vi "motorJoystickcore.vi"(4 "button info":T2, 6 "axis info":T1, 8 "error in":errorcluster[](array[cluster]), 9 "Motor Limits":T3, 10 "Array in":refnum<k7>[](array[refnum]), 11 "Motor serial numbers":i32[](array[numeric])) -> (0 "error out":errorcluster[](array[cluster]), 2 "XYZ position":sgl[](array[numeric]))   [LabVIEW 2014]
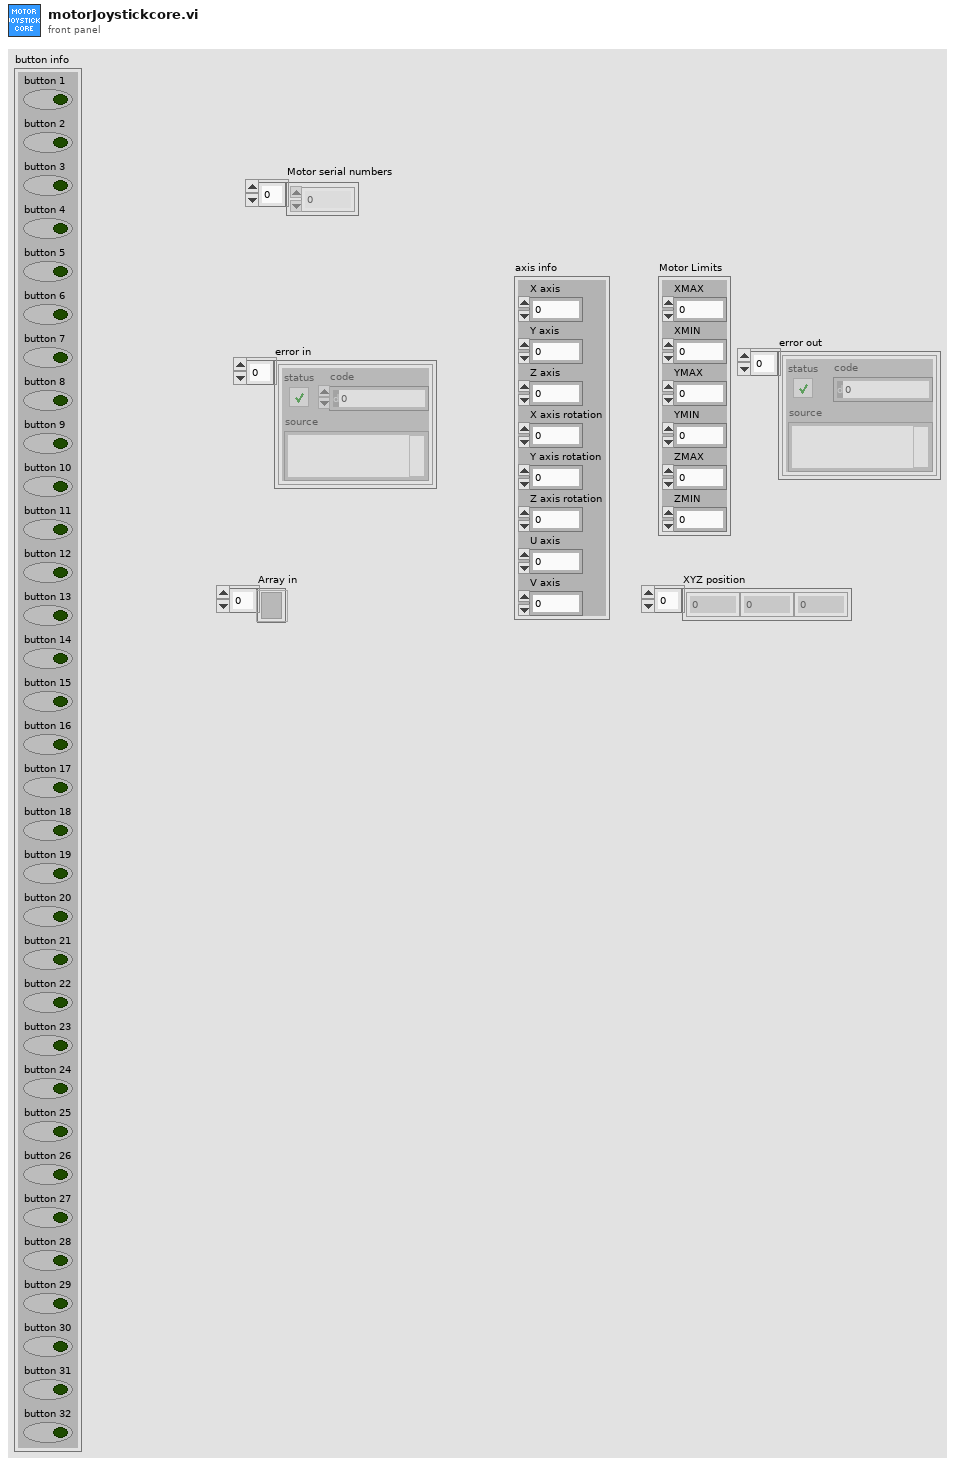
[diagram p1: front panel]
types:
  T1 = cluster{"X axis":i32, "Y axis":i32, "Z axis":i32, "X axis rotation":i32, "Y axis rotation":i32, "Z axis rotation":i32, "U axis":i32, "V axis":i32}
  T2 = cluster{"button 1":bool, "button 2":bool, "button 3":bool, "button 4":bool, "button 5":bool, "button 6":bool, "button 7":bool, "button 8":bool, "button 9":bool, "button 10":bool, "button 11":bool, "button 12":bool, "button 13":bool, "button 14":bool, "button 15":bool, "button 16":bool, "button 17":bool, "button 18":bool, "button 19":bool, "button 20":bool, "button 21":bool, "button 22":bool, "button 23":bool, "button 24":bool, "button 25":bool, "button 26":bool, "button 27":bool, "button 28":bool, "button 29":bool, "button 30":bool, "button 31":bool, "button 32":bool}
  T3 = cluster{"XMAX":sgl, "XMIN":sgl, "YMAX":sgl, "YMIN":sgl, "ZMAX":sgl, "ZMIN":sgl}
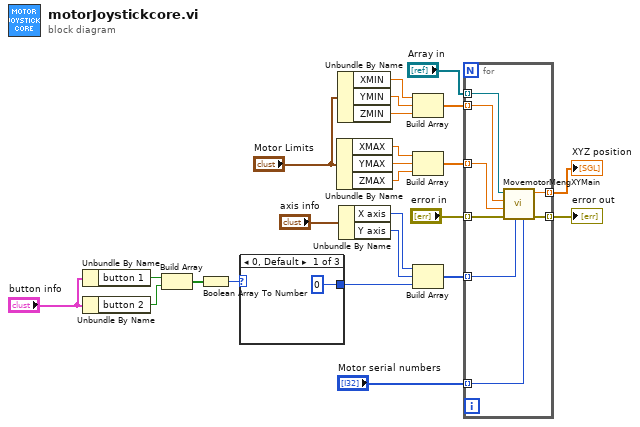
[diagram p0: block diagram]
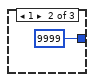
[diagram p2: hidden frame]
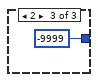
[diagram p3: hidden frame]
diagram:
  n1 = Unbundle By Name("button info") -> ("button 1"=w20:bool)
  n2 = Unbundle By Name("button info") -> ("button 2"=w21:bool)
  n3 = Build Array(w20, w21) -> (w22:bool[])
  n4 = Boolean Array To Number(Boolean array=w22) -> (number=w23:u32)
  n5 = case shown="0, Default" w23 {
    tunnel: [0 ("Y axis") 9999 ("Y axis") -9999 ("Y axis")] -> w11
    frame 0, Default {
    }
    frame 1 {
    }
    frame 2 {
    }
  }
  n6 = Unbundle By Name("Motor Limits") -> ("XMAX"=w19:sgl, "YMAX"=w18:sgl, "ZMAX"=w17:sgl)
  n7 = Unbundle By Name("Motor Limits") -> ("XMIN"=w14:sgl, "YMIN"=w15:sgl, "ZMIN"=w13:sgl)
  n8 = Unbundle By Name("axis info") -> ("X axis"=w10:i32, "Y axis"=w9:i32)
  n9 = Build Array(w14, w15, w13) -> (w8:sgl[])
  n10 = Build Array(w19, w18, w17) -> (w7:sgl[])
  n11 = Build Array(w10, w9, w11) -> (w3:i32[])
  n12 = for {
    tunnel: w8 -> [w35] mode=indexing
    tunnel: w7 -> [w34] mode=indexing
    tunnel: "Array in" -> [w33] mode=indexing
    tunnel: "error in" -> [w32] mode=indexing
    tunnel: [w31] -> w4 mode=indexing
    tunnel: w3 -> [w30] mode=indexing
    tunnel: [w29] -> w2 mode=indexing
    tunnel: "Motor serial numbers" -> [w28] mode=indexing
    n13 = call "MovemotorMengXYMain.vi"("Serial number"=w28, "Joystick axis"=w30, "error in (no error)"=w32, "MAX"=w34, "MIN"=w35, "Automation Refnum in"=w33) -> ("error out"=w29:errorcluster, "XorYPosition"=w31:sgl)  [unwired: 3 in, 1 out]
  }
  "error out" <- w2
  "XYZ position" <- w4
